vi "simultion_time_MRC.vi"() -> ()   [LabVIEW 2014]
uses:
  <vilib>/addons/Modulation/Digital/General/MT Generate Bits (Galois, PN Order).vi
  <vilib>/addons/Modulation/Digital/Support/Common/Validators/mod_Generate Bits Validate.vi
  <vilib>/addons/Modulation/Analog/support/mod_Set Error Source.vi
  <vilib>/addons/Modulation/Digital/General/subVIs/mod_Generate Bits PN Sequence.vi
  <vilib>/addons/Modulation/Digital/General/MT Generate QAM System Parameters(M).vi
  <vilib>/addons/Modulation/Digital/General/MT Map Bits to QAM Symbols.vi
  <vilib>/addons/Modulation/Digital/Support/Common/Validators/mod_Generate Filter Coefficients Validate.vi
  <vilib>/addons/Modulation/Digital/General/subVIs/mod_Generate Filter Coefficients.vi
  <vilib>/addons/Modulation/Digital/General/MT Apply Pulse Shaping Filter (Generic).vi
  <vilib>/addons/Modulation/Digital/General/MT Apply Matched Filter (Generic).vi
  <vilib>/addons/Modulation/Digital/General/MT Align to Ideal Symbols (Generic).vi
  <vilib>/addons/Modulation/Digital/General/MT Map QAM Symbols to Bits.vi
  <vilib>/addons/Modulation/niDMT.lvlib
panel:
  out "Waveform Chart":dbl[](graph)
  in  "IQ Rate":dbl=1000000.0 format="%#_6p"
  out "output bit stream":i8[](array[numeric])
  out "sum":i16
  out "size(s)":i32
  out "input bits stream":i8[](array[numeric]) caption="input bit stream"
  in  "CP length":u32=32 caption="CP Size"
  in  "Message Carrier":u32=128
  in  "FFT Size":u32=256
  in  "M-QAM (16)":i32=16
  in  "total bits (128)":i32=512 caption="total bits (512)"
  in  "samples per symbol (16)":i32=4
  in  "pulse shaping filter (none)":T1(ring)=enum."Raised Cosine"
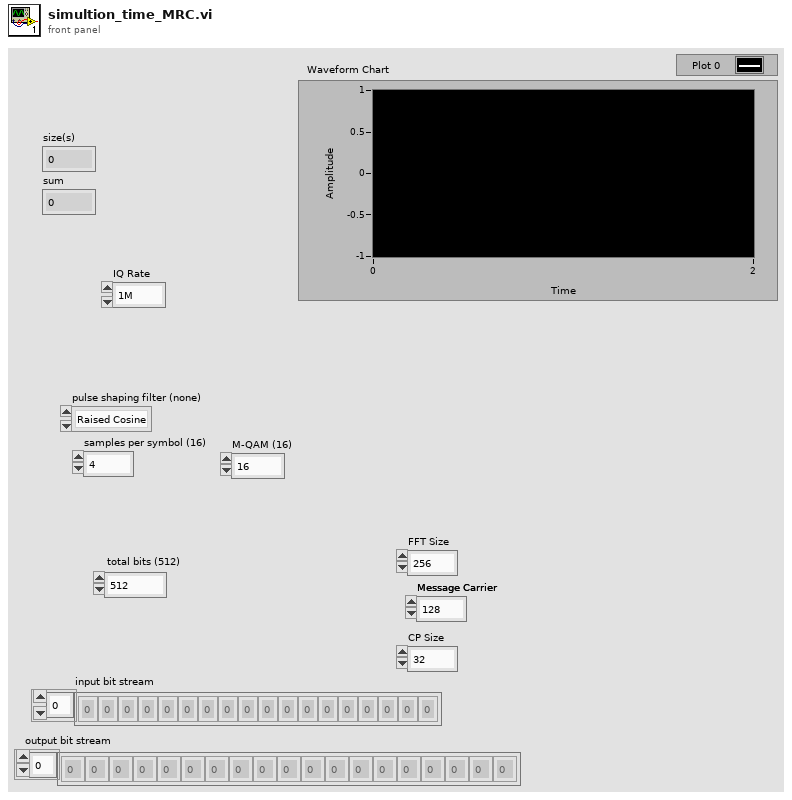
[diagram p1: front panel]
types:
  T1 = enum16{"none", "Raised Cosine", "Root Raised Cos", "Gaussian"}
  T2 = enum16{"FSK", "PSK", "QAM", "MSK", "PAM", "ASK", "CPM"}
  T3 = cluster{"samples per symbol (16)":i32, "symbol map":cdb[]}
  T4 = typedef "niAMT.lvlib/Complex Data Waveform.ctl" = cluster{"t0":dbl, "dt":dbl, "Y":cdb[]}
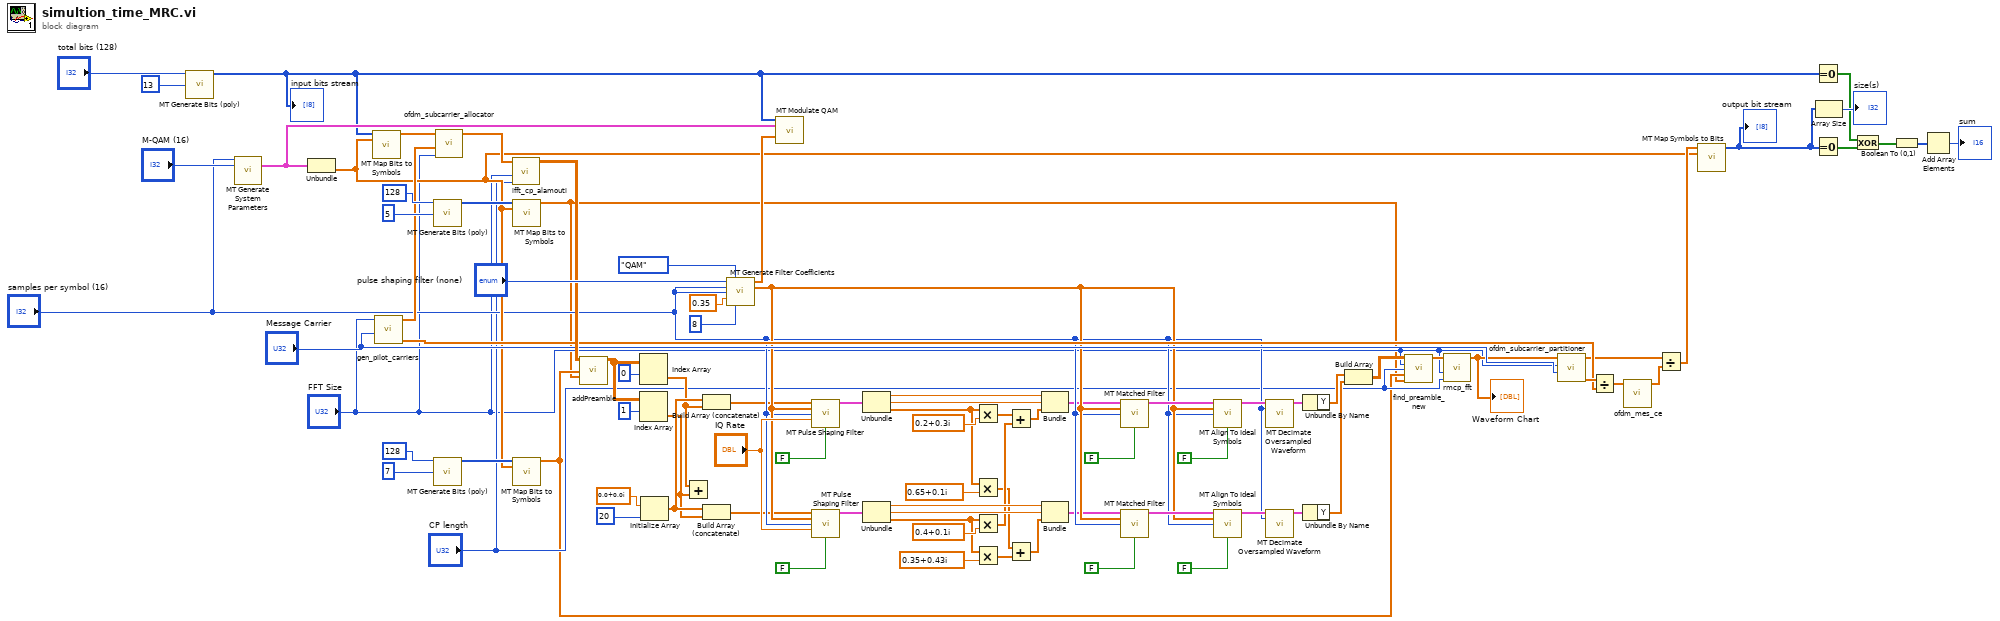
[diagram p0: block diagram]
diagram:
  n1 = call-poly <vilib>:"MT Generate Bits (poly).vi"("total bits (128)"="total bits (128)", "PN sequence order (9)"=13) -> ("output bit stream"=w59:i8[])  [unwired: 11 in, 2 out]
  "input bits stream" <- w59
  n2 = call-poly <vilib>:"MT Generate System Parameters.vi"("samples per symbol (16)"="samples per symbol (16)", "M-QAM (16)"="M-QAM (16)") -> ("QAM system parameters"=w80:T3)  [unwired: 11 in, 2 out]
  n3 = Unbundle(w80) -> ("symbol map"=w64:cdb[])  [unwired: 1 out]
  n4 = call-poly <vilib>:"MT Map Bits to Symbols.vi"("input bit stream"=w59, "symbol map"=w64) -> ("symbols"=w77:cdb[])  [unwired: 12 in, 1 out]
  n5 = call "gen_pilot_carriers.vi"("message carrier"="Message Carrier", "FFT size"="FFT Size") -> ("RX pilot carriers"=w68:cdb[], "TX pilot carriers"=w76:cdb[])  [unwired: 8 in]
  n6 = call-poly <vilib>:"MT Generate Bits (poly).vi"("total bits (128)"=128, "PN sequence order (9)"=5) -> ("output bit stream"=w74:i8[])  [unwired: 11 in, 2 out]
  n7 = call-poly <vilib>:"MT Generate Bits (poly).vi"("total bits (128)"=128, "PN sequence order (9)"=7) -> ("output bit stream"=w75:i8[])  [unwired: 11 in, 2 out]
  n8 = call "ofdm_subcarrier_allocator.vi"("fft size"="FFT Size", "pilot symbol"=w76, "message symbol"=w77) -> ("OFDM symbol"=w84:cdb[])  [unwired: 8 in]
  n9 = call "ifft_cp_alamouti.vi"("CP Length"="CP length", "FFT Size"="FFT Size", "Modulated Stream"=w84) -> ("Baseband Streams"=w82:cdb[][])  [unwired: 8 in]
  n10 = call-poly <vilib>:"MT Map Bits to Symbols.vi"("input bit stream"=w74, "symbol map"=w64) -> ("symbols"=w1:cdb[])  [unwired: 12 in, 1 out]
  n11 = call-poly <vilib>:"MT Map Bits to Symbols.vi"("input bit stream"=w75, "symbol map"=w64) -> ("symbols"=w2:cdb[])  [unwired: 12 in, 1 out]
  n12 = call "addPreamble.vi"("Input Symbol Stream"=w82, "Training Sequence"=w2, "Training Sequence 2"=w1) -> ("Output Transmit \nPackets"=w62:cdb[][])  [unwired: 11 in, 1 out]
  n13 = Index Array(array=w62, index (row)=0) -> (element=w30:cdb[])  [unwired: 1 in]
  n14 = Index Array(array=w62, index (row)=1) -> (element=w29:cdb[])  [unwired: 1 in]
  n15 = Initialize Array(cdb 0.0+0.0i ("element"), 20 ("dimension size")) -> (w31:cdb[])
  n16 = Add(x=w30, y=w29) -> ()  [unwired: 1 out]
  n17 = Build Array (concatenate)(w31, w30) -> (w33:cdb[])
  n18 = Build Array (concatenate)(w31, w29) -> (w32:cdb[])
  n19 = call <vilib>:"MT Generate Filter Coefficients.vi"("pulse shaping filter (none)"="pulse shaping filter (none)", "modulation type"=T2."QAM", "pulse shaping samples per symbol (16)"="samples per symbol (16)", "matched samples per symbol (16)"="samples per symbol (16)", "filter parameter"=0.35, "filter length (symbols)"=8) -> ("pulse shaping filter coefficients"=w78:dbl[], "matched filter coefficients"=w46:dbl[])  [unwired: 7 in, 1 out]
  n20 = call <vilib>:"MT Modulate QAM.vi"("input bit stream"=w59, "QAM system parameters"=w80, "pulse shaping filter coefficients"=w78) -> ()  [unwired: 10 in, 3 out]
  n21 = call-poly <vilib>:"MT Pulse Shaping Filter.vi"("symbols"=w33, "pulse shaping filter coefficients"=w46, "samples per symbol (16)"="samples per symbol (16)", "symbol rate (Hz)"="IQ Rate", "reset? (T)"=FALSE) -> ("output complex waveform"=w26:T4)  [unwired: 9 in, 1 out]
  n22 = call-poly <vilib>:"MT Pulse Shaping Filter.vi"("symbols"=w32, "pulse shaping filter coefficients"=w46, "samples per symbol (16)"="samples per symbol (16)", "symbol rate (Hz)"="IQ Rate", "reset? (T)"=FALSE) -> ("output complex waveform"=w22:T4)  [unwired: 9 in, 1 out]
  n23 = Unbundle(w26) -> ("t0"=w25:dbl, "dt"=w24:dbl, "Y"=w15:cdb[])
  n24 = Unbundle(w22) -> ("t0"=w21:dbl, "dt"=w20:dbl, "Y"=w14:cdb[])
  n25 = Multiply(x=w15, y=cdb 0.2+0.3i) -> (x*y=w18:cdb[])
  n26 = Multiply(x=w15, y=cdb 0.65+0.1i) -> (x*y=w11:cdb[])
  n27 = Multiply(x=w14, y=cdb 0.4+0.1i) -> (x*y=w17:cdb[])
  n28 = Multiply(x=w14, y=cdb 0.35+0.43i) -> (x*y=w10:cdb[])
  n29 = Add(x=w18, y=w17) -> (x+y=w16:cdb[])
  n30 = Add(x=w11, y=w10) -> (x+y=w9:cdb[])
  n31 = Bundle("t0"=w25, "dt"=w24, w16) -> (w23:cluster{"t0":dbl, "dt":dbl, cdb[]})  [unwired: 1 in]
  n32 = Bundle("t0"=w21, "dt"=w20, w9) -> (w19:cluster{"t0":dbl, "dt":dbl, cdb[]})  [unwired: 1 in]
  n33 = call-poly <vilib>:"MT Matched Filter.vi"("input complex waveform"=w23, "matched filter coefficients"=w46, "samples per symbol (16)"="samples per symbol (16)", "reset? (T)"=FALSE) -> ("output complex waveform"=w52:T4)  [unwired: 10 in, 1 out]
  n34 = call-poly <vilib>:"MT Matched Filter.vi"("input complex waveform"=w19, "matched filter coefficients"=w46, "samples per symbol (16)"="samples per symbol (16)", "reset? (T)"=FALSE) -> ("output complex waveform"=w50:T4)  [unwired: 10 in, 1 out]
  n35 = call-poly <vilib>:"MT Align To Ideal Symbols.vi"("input complex waveform"=w52, "matched filter coefficients"=w46, "samples per symbol (16)"="samples per symbol (16)", "reset? (T)"=FALSE) -> ("output complex waveform"=w51:T4)  [unwired: 9 in, 2 out]
  n36 = call-poly <vilib>:"MT Align To Ideal Symbols.vi"("input complex waveform"=w50, "matched filter coefficients"=w46, "samples per symbol (16)"="samples per symbol (16)", "reset? (T)"=FALSE) -> ("output complex waveform"=w49:T4)  [unwired: 9 in, 2 out]
  n37 = call <vilib>:"MT Decimate Oversampled Waveform.vi"("input complex waveform"=w51, "decimation factor"="samples per symbol (16)") -> ("output complex waveform"=w48:T4)  [unwired: 12 in, 1 out]
  n38 = call <vilib>:"MT Decimate Oversampled Waveform.vi"("input complex waveform"=w49, "decimation factor"="samples per symbol (16)") -> ("output complex waveform"=w47:T4)  [unwired: 12 in, 1 out]
  n39 = Unbundle By Name(w48) -> ("Y"=w8:cdb[])
  n40 = Unbundle By Name(w47) -> ("Y"=w7:cdb[])
  n41 = Build Array(w8, w7) -> (w6:cdb[][])
  n42 = call "find_preamble_new.vi"("received \ntime symbol"=w6, "FFT Size"="FFT Size", "CP Length"="CP length", "1st preamble"=w2, "2nd preamble"=w1) -> ("Received OFDM Symbol"=w5:cdb[])  [unwired: 10 in]
  n43 = call "rmcp_fft.vi"("CP length"="CP length", "fft size"="FFT Size", "time symbol"=w5) -> ("freq output"=w36:cdb[])  [unwired: 8 in]
  "Waveform Chart" <- w36
  n44 = call "ofdm_subcarrier_partitioner.vi"("message carrier"="Message Carrier", "FFT size"="FFT Size", "received symbol"=w36) -> ("pilot subcarriers"=w71:cdb[], "message subcarriers"=w66:cdb[])  [unwired: 7 in]
  n45 = Divide(x=w71, y=w68) -> (x/y=w70:cdb[])
  n46 = call "ofdm_mes_ce.vi"("ZF \nchannel \nestimates"=w70) -> ("interpolated\n mes carrier CE"=w67:cdb[])  [unwired: 10 in]
  n47 = Divide(x=w66, y=w67) -> (x/y=w65:cdb[])
  n48 = call-poly <vilib>:"MT Map Symbols to Bits.vi"("symbols"=w65, "symbol map"=w64) -> ("output bit stream"=w60:i8[])  [unwired: 12 in, 1 out]
  "output bit stream" <- w60
  n49 = Equal To 0?(x=w59) -> (x = 0?=w57:bool[])
  n50 = Equal To 0?(x=w60) -> (x = 0?=w58:bool[])
  n51 = Array Size(array=w60) -> (size(s)=→"size(s)":i32)
  n52 = Exclusive Or(1:w58, 2:w57) -> (0:w56:bool[])
  n53 = Boolean To (0,1)(Boolean=w56) -> (0, 1=w55:i16[])
  n54 = Add Array Elements(numeric array=w55) -> (sum=→"sum":i16)
